vi "readFromXML.vi"(8 "error in (no error)":errorcluster, 10 "XML in":string, 11 "CollOffset in":refnum<class "CollOffset.lvclass">) -> (0 "error out":errorcluster, 3 "CollOffset out":refnum<class "CollOffset.lvclass">)   [LabVIEW 2022 SP3, in "TCSDataDefinitions.lvlib" / "TCSCommand.lvlib" / "OffsetCommands.lvlib" / "CollOffset.lvclass"]
uses:
  CollOffset.lvclass
  <userlib>/Common/UnitsAndXML/FlattenItemWithUnitToXML/FlattenPlaneAngleToXML/PlaneAngleUnit.ctl
  CollOffset.lvclass/CollOffset.ctl
  CollimationOffsetCommands/CollimationOffsetCommands.lvclass
  <userlib>/Common/UnitsAndXML/UnitsAndXML.lvlib
  <userlib>/Common/XML/XMLParser/XMLParser.lvclass
panel:
  out "ce":dbl[unit]
  out "ca":dbl[unit]
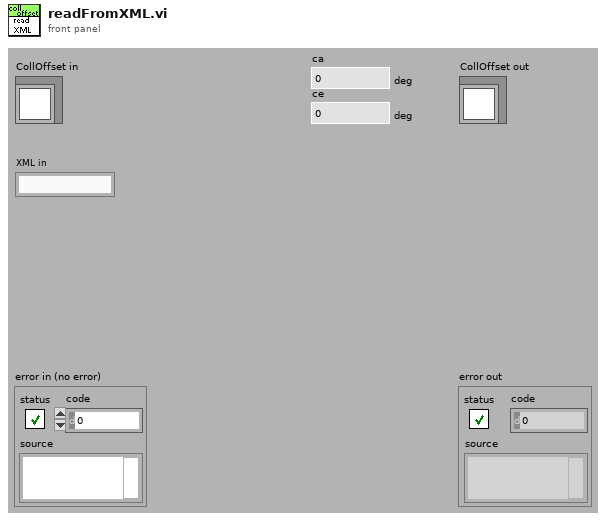
[diagram p1: front panel]
types:
  T1 = typedef "UnitsAndXML.lvlib/PlaneAngleUnit.ctl" = enum16{"rad", "deg", "'", "\""}
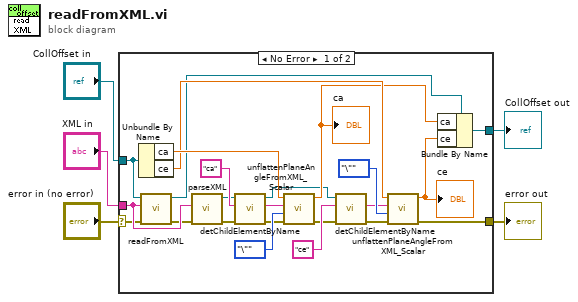
[diagram p0: block diagram]
diagram:
  n1 = case shown="No Error" "error in (no error)" {
    selector: "error in (no error)" -> [w23 w30]
    tunnel: [w9 w30] -> w4
    tunnel: [w12 w29] -> w2
    tunnel: "CollOffset in" -> [w13 w29]
    tunnel: "XML in" -> [w28 _]
    frame No Error {
      n2 = Unbundle By Name(w13) -> ("ca"=w22:dbl[unit], "ce"=w19:dbl[unit])
      n3 = call-parent "readFromXML.vi"("error in (no error)"=w23, "XML in"=w28, "CollimationOffsetCommands in"=w13) -> ("error out"=w27:errorcluster, "CollimationOffsetCommands out"=w8:refnum<class "CollOffset.lvclass">)  [unwired: 7 out]
      n4 = call <userlib>:"parseXML.vi"("error in (no error)"=w27, "XMLString in"=w28) -> ("error out"=w26:errorcluster, "Element out"=w7:refnum<class "XMLParser.lvclass">)  [unwired: 8 in]
      n5 = call <userlib>:"detChildElementByName.vi"("error in (no error)"=w26, "childName"="ca" ("ChildName"), "Element in"=w7) -> ("error out"=w18:errorcluster, "childXML"=w21:string, "Element out"=w6:refnum<class "XMLParser.lvclass">)  [unwired: 5 in, 1 out]
      n6 = call <userlib>:"unflattenPlaneAngleFromXML_Scalar.vi"("error in (no error)"=w18, "planeAngleUnitInXML"=PlaneAngleUnit."\"", "xmlString"=w21, "planeAngleForType"=w22) -> ("error out"=w17:errorcluster, "planeAngle"=w10:dbl[unit])  [unwired: 6 in]
      "ca" <- w10
      n7 = call <userlib>:"detChildElementByName.vi"("error in (no error)"=w17, "childName"="ce" ("ChildName"), "Element in"=w6) -> ("error out"=w16:errorcluster, "childXML"=w14:string)  [unwired: 5 in, 2 out]
      n8 = call <userlib>:"unflattenPlaneAngleFromXML_Scalar.vi"("error in (no error)"=w16, "planeAngleUnitInXML"=PlaneAngleUnit."\"", "xmlString"=w14, "planeAngleForType"=w19) -> ("error out"=w9:errorcluster, "planeAngle"=w11:dbl[unit])  [unwired: 6 in]
      "ce" <- w11
      n9 = Bundle By Name(cluster=w8, "ca"=w10, "ce"=w11) -> (w12:refnum<class "CollOffset.lvclass">)
    }
    frame Error {
    }
  }
  "error out" <- w4
  "CollOffset out" <- w2
